vi "Read_Param.vi"(6 "Énum":enum16{"STR", "DBL", "U32", "chemin"}(ring), 8 "errin":errorcluster, 10 "section":string, 11 "key":string caption="clé") -> (0 "error out":errorcluster, 1 "U32":u32, 2 "str":string, 3 "dbl":dbl, 4 "value":path)   [LabVIEW 2020]
uses:
  <vilib>/Utility/config.llb/Read Key (String).vi
  <vilib>/Utility/config.llb/Read Key (Path).vi
  <vilib>/Utility/config.llb/Read Key (U32).vi
  <vilib>/Utility/config.llb/Read Key (Double).vi
  <vilib>/Utility/config.llb/NI_LVConfig.lvlib
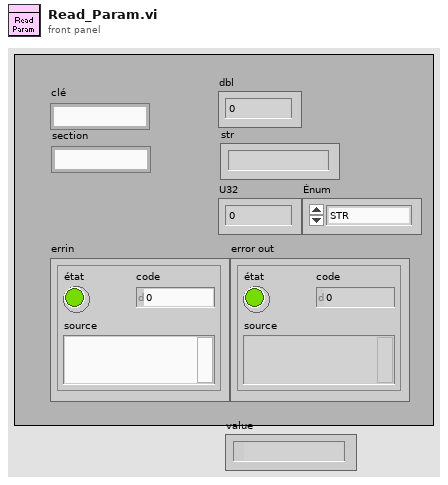
[diagram p1: front panel]
types:
  T1 = typedef "NI_LVConfig.lvlib/Config Data RefNum.ctl" = refnum<k1>
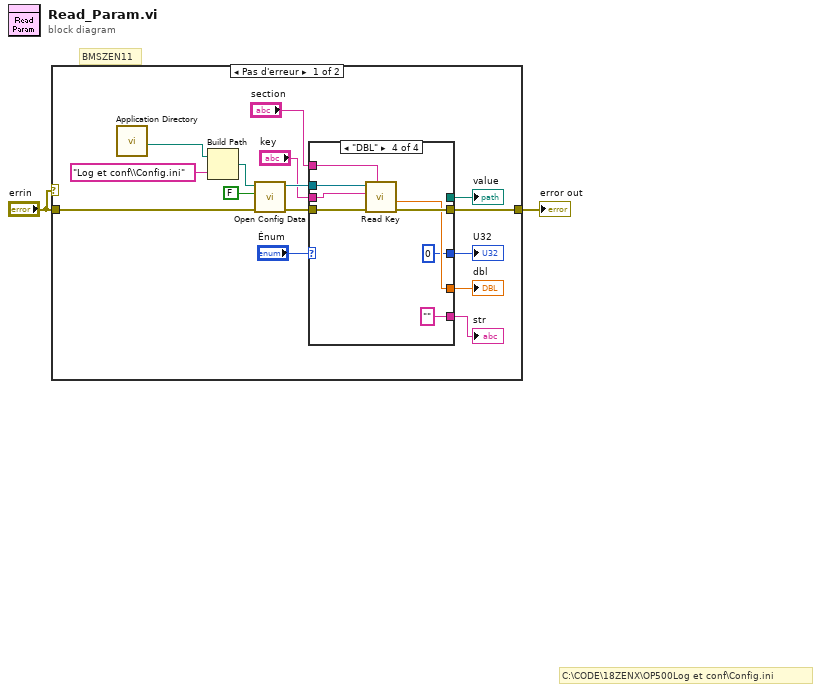
[diagram p0: block diagram]
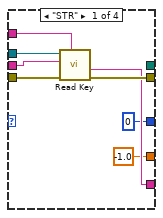
[diagram p2: hidden frame]
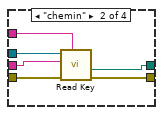
[diagram p3: hidden frame]
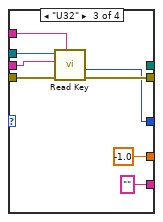
[diagram p4: hidden frame]
diagram:
  # "C:\\CODE\\18ZENX\\OP500Log et conf\\Config.ini"
  # "BMSZEN11"
  n1 = case shown="Pas d'erreur" "errin" {
    tunnel: "errin" -> [w14 w48]
    tunnel: [w9 w48] -> w2
    frame No Error {
      n2 = call <vilib>:"Application Directory.vi"() -> ("Application Directory"=w3:path)
      n3 = Build Path(base path=w3, name or relative path="Log et conf\\Config.ini") -> (appended path=w16:path)
      n4 = call <vilib>:"Open Config Data.vi"("error in (no error)"=w14, "create file if necessary (T)"=FALSE, "configuration file path"=w16) -> ("error out"=w13:errorcluster, "refnum"=w12:T1)  [unwired: 6 in, 1 out]
      n5 = case shown="\"DBL\"" "Énum" {
        tunnel: w13 -> [w25 w31 w39 w47]
        tunnel: w12 -> [w24 w29 w38 w46]
        tunnel: "section" -> [w23 w26 w37 w45]
        tunnel: "key" -> [w22 w28 w36 w44]
        tunnel: [w21 w30 w35 w43] -> w9
        tunnel: [-1.0 ("value") _ -1.0 ("value") w42] -> w8
        tunnel: [w20 _ "" ("value") "" ("value")] -> w7
        tunnel: [u32 0 ("value") _ w32 u32 0 ("value")] -> w6
        tunnel: [_ w27 _ _] -> w4
        frame "STR" {
          n6 = call-poly <vilib>:"Read Key.vi"("section"=w23, "error in (no error)"=w25, "key"=w22, "refnum"=w24) -> ("error out"=w21:errorcluster, "value"=w20:string)  [unwired: 4 in, 2 out]
        }
        frame "chemin" {
          n7 = call-poly <vilib>:"Read Key.vi"("section"=w26, "error in (no error)"=w31, "key"=w28, "refnum"=w29) -> ("error out"=w30:errorcluster, "value"=w27:path)  [unwired: 4 in, 2 out]
        }
        frame "U32" {
          n8 = call-poly <vilib>:"Read Key.vi"("section"=w37, "error in (no error)"=w39, "key"=w36, "refnum"=w38) -> ("error out"=w35:errorcluster, "value"=w32:u32)  [unwired: 4 in, 2 out]
        }
        frame "DBL" {
          n9 = call-poly <vilib>:"Read Key.vi"("section"=w45, "error in (no error)"=w47, "key"=w44, "refnum"=w46) -> ("error out"=w43:errorcluster, "value"=w42:dbl)  [unwired: 4 in, 2 out]
        }
      }
      "dbl" <- w8
      "str" <- w7
      "U32" <- w6
      "value" <- w4
    }
    frame Error {
    }
  }
  "error out" <- w2
